vi "Right-Click Menu.vi"(6 "State In":T2={"Worker Library Path"=path "", "Block Label"="", "Types"=[], "Selections"=[], "Icon"={"image type"=0, "image depth"=0, "image"=[], "mask"=[], "colors"=[], "Rectangle"={"left"=0, "top"=0, "right"=0, "bottom"=0}}, "Errors"={"Terminals"=[], "Generate"={"status"=FALSE, "code"=0, "source"=""}, "General"={"status"=FALSE, "code"=0, "source"=""}}, "Calculated Sizes"={"Block Width"=0, "Block Height"=0, "Half Width"=0, "Icon Top"=0, "Icon Bottom"=0, "Label Width"=0, "Half Label"=0, "Label Top"=0, "Text Width"=0, "Half Text"=0, "Text Height"=0, "Label Height"=0, "Expanded Width"=0, "Label Bottom"=0, "Expanded Top"=0, "Expanded Bottom"=0, "Expanded Height"=0, "Min Height"=0, "Max Height"=0}, "Special Terminal Indices"={"Action"=-1, "Init"=-1, "Tag"=-1, "State in"=-1, "State out"=-1, "Error"=-1, "Control"=-1, "Config"=-1}, "Terminals"=[], "Temp VI Name"="", "Description"="", "Smol Mode"=FALSE}, 10 "Point":T14, 11 "MenuRef in":T1) -> (0 "error out":errorcluster, 3 "MenuRef":T1)   [LabVIEW 2022 SP3, in "FlexBlocks Support.lvlib"]
uses:
  FlexBlocks Support.lvlib
  <vilib>/XNodeSupport/XNodeMenuRef.ctl
  <vilib>/XNodeSupport/XNodePoint.ctl
  <vilib>/XNodeSupport/XNodeInt.ctl
  Flex Block/State.ctl
  Type Descriptor.ctl
  Terminal Direction.ctl
  Value Mode.ctl
  Special Terminal.ctl
  <vilib>/picture/picture.llb/imagedata.ctl
  XNode Errors.ctl
  Calculated Sizes.ctl
  Special Terminal Indices.ctl
  Terminal Status.ctl
  Terminal State.ctl
  Terminal Draw Style.ctl
  Menu Tag.ctl
  <vilib>/XNodeSupport/NI_XNodeSupport.lvlib
  Flex Block/Flex Block.xnode
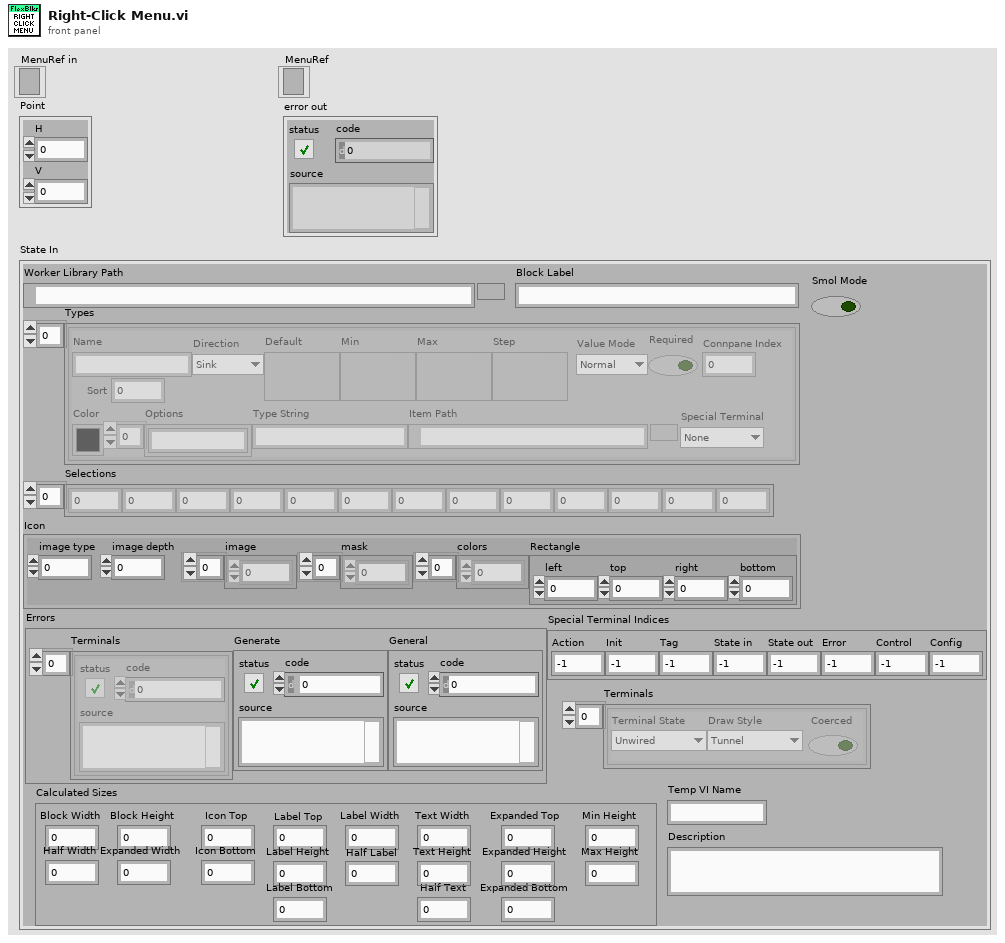
[diagram p1: front panel]
types:
  T1 = typedef "NI_XNodeSupport.lvlib/XNodeMenuRef.ctl" = refnum<k9>
  T2 = typedef "Flex Block.xnode/State.ctl" = cluster{"Worker Library Path":path, "Block Label":string, "Types":T3[], "Selections":i32[], "Icon":T7, "Errors":T8, "Calculated Sizes":T9, "Special Terminal Indices":T10, "Terminals":T11[], "Temp VI Name":string, "Description":string, "Smol Mode":bool}
  T3 = typedef "FlexBlocks Support.lvlib/Type Descriptor.ctl" = cluster{"Name":string, "Direction":T4, "Default":variant, "Min":variant, "Max":variant, "Step":variant, "Value Mode":T5, "Color":u32, "Options":string[], "Type String":string, "Item Path":path, "Required":bool, "Connpane Index":i32, "Special Terminal":T6, "Sort":i32}
  T4 = typedef "FlexBlocks Support.lvlib/Terminal Direction.ctl" = enum16{"Sink", "Source"}
  T5 = typedef "FlexBlocks Support.lvlib/Value Mode.ctl" = enum16{"Normal", "Range", "Select"}
  T6 = typedef "FlexBlocks Support.lvlib/Special Terminal.ctl" = enum16{"None", "Action", "Init", "Tag", "State in", "State out", "Error", "Control", "Config"}
  T7 = typedef "imagedata.ctl" = cluster{"image type":i32, "image depth":i32, "image":u8[], "mask":u8[], "colors":u32[], "Rectangle":cluster{"left":i16, "top":i16, "right":i16, "bottom":i16}}
  T8 = typedef "FlexBlocks Support.lvlib/XNode Errors.ctl" = cluster{"Terminals":errorcluster[], "Generate":errorcluster, "General":errorcluster}
  T9 = typedef "FlexBlocks Support.lvlib/Calculated Sizes.ctl" = cluster{"Block Width":i32, "Block Height":i32, "Half Width":i32, "Icon Top":i32, "Icon Bottom":i32, "Label Width":i32, "Half Label":i32, "Label Top":i32, "Text Width":i32, "Half Text":i32, "Text Height":i32, "Label Height":i32, "Expanded Width":i32, "Label Bottom":i32, "Expanded Top":i32, "Expanded Bottom":i32, "Expanded Height":i32, "Min Height":i32, "Max Height":i32}
  T10 = typedef "FlexBlocks Support.lvlib/Special Terminal Indices.ctl" = cluster{"Action":i32, "Init":i32, "Tag":i32, "State in":i32, "State out":i32, "Error":i32, "Control":i32, "Config":i32}
  T11 = typedef "FlexBlocks Support.lvlib/Terminal Status.ctl" = cluster{"Terminal State":T12, "Draw Style":T13, "Coerced":bool}
  T12 = typedef "FlexBlocks Support.lvlib/Terminal State.ctl" = enum16{"Unwired", "BadType", "BadRef", "Channel", "Value", "Control Ref"}
  T13 = typedef "FlexBlocks Support.lvlib/Terminal Draw Style.ctl" = enum16{"Tunnel", "BadType", "BadRef", "Channel", "Value", "Control Ref"}
  T14 = typedef "NI_XNodeSupport.lvlib/XNodePoint.ctl" = cluster{"H":T15, "V":T15}
  T15 = typedef "NI_XNodeSupport.lvlib/XNodeInt.ctl" = i32
  T16 = typedef "FlexBlocks Support.lvlib/Right-Click Menu Target.ctl" = enum16{"Frame", "Label", "Value", "Terminal", "Icon"}
  T17 = typedef "FlexBlocks Support.lvlib/Menu Tag.ctl" = enum16{"Unknown", "Create Channel Writer", "Create Lossy Reader", "Create Lossless Reader", "Create Event Reader", "Smol Mode", "Open Block VI", "Open Block Library"}
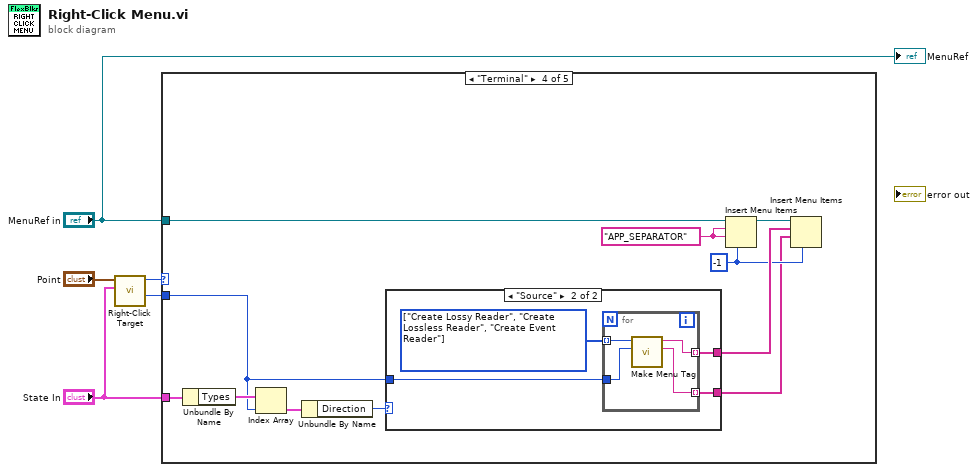
[diagram p0: block diagram]
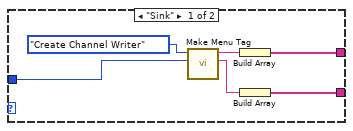
[diagram p5: hidden frame]
diagram:
  n1 = call "Right-Click Target.vi"("State In"="State In", "Point"="Point") -> ("Target Index"=w2:i32, "Menu Target"=w4:T16)  [unwired: 8 in]
  n2 = case shown="\"Terminal\"" w4 {
    tunnel: w2 -> [_ _ _ w7 _]
    tunnel: "State In" -> [_ _ _ w16 _]
    tunnel: "MenuRef in" -> [_ _ _ w10 _]
    frame "Frame" {
    }
    frame "Label" {
    }
    frame "Value" {
    }
    frame "Terminal" {
      w9 = "APP_SEPARATOR"
      w8 = -1
      n3 = Unbundle By Name(w16) -> ("Types"=w15:T3[])
      n4 = Index Array(array=w15, index=w7) -> (element=w14:T3)
      n5 = Unbundle By Name(w14) -> ("Direction"=w13:T4)
      n6 = case shown="\"Source\"" w13 {
        tunnel: [w19 w24] -> w12
        tunnel: w7 -> [w22 w25]
        tunnel: [w17 w23] -> w6
        frame "Sink" {
          n7 = call "Make Menu Tag.vi"("Int"=w22, "Menu Tag"=Menu_Tag."Create Channel Writer") -> ("Tag String"=w18:string, "Label"=w20:string)  [unwired: 8 in]
          n8 = Build Array(w20) -> (w19:string[])
          n9 = Build Array(w18) -> (w17:string[])
        }
        frame "Source" {
          w26 = T17[] [enum."Create Lossy Reader", enum."Create Lossless Reader", enum."Create Event Reader"] items=["Unknown", "Create Channel Writer", "Create Lossy Reader", "Create Lossless Reader", "Create Event Reader", "Smol Mode", "Open Block VI", "Open Block Library"]
          n10 = for {
            tunnel: w26 -> [w30] mode=indexing
            tunnel: w25 -> [w29]
            tunnel: [w28] -> w24 mode=indexing
            tunnel: [w27] -> w23 mode=indexing
            n11 = call "Make Menu Tag.vi"("Int"=w29, "Menu Tag"=w30) -> ("Tag String"=w27:string, "Label"=w28:string)  [unwired: 8 in]
          }
        }
      }
      n12 = Insert Menu Items(4:w8, 7:w9, 8:w9, 9:w10) -> (3:w11:refnum<k9>)  [unwired: 2 in, 2 out]
      n13 = Insert Menu Items(4:w8, 7:w6, 8:w12, 9:w11) -> ()  [unwired: 2 in, 3 out]
    }
    frame "Icon" {
    }
  }
  "MenuRef" <- "MenuRef in"
